vi "Remove Device.vi"(8 "error in (no error)":errorcluster, 10 "Key":T1, 11 "DeviceListPanel in":refnum<class "DeviceListPanel.lvclass">) -> (0 "error out":errorcluster, 3 "DeviceListPanel out":refnum<class "DeviceListPanel.lvclass">)   [LabVIEW 2020, in "PicoG-App.lvlib" / "DeviceListPanel.lvclass"]
uses:
  DeviceListPanel.lvclass
  DeviceListPanel.lvclass/DeviceListPanel.ctl
  Device/Device Key.ctl
  Device/Device.lvclass
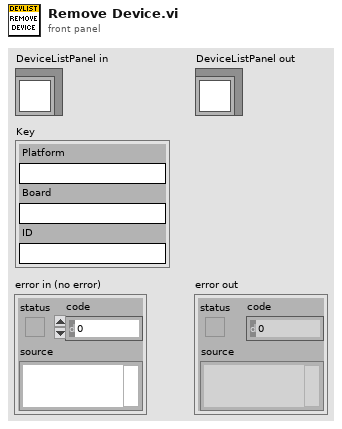
[diagram p1: front panel]
types:
  T1 = typedef "PicoG-App.lvlib/Device.lvclass/Device Key.ctl" = cluster{"Platform":string, "Board":string, "ID":string}
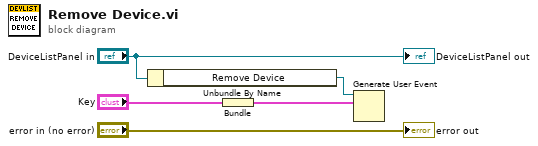
[diagram p0: block diagram]
diagram:
  n1 = Unbundle By Name("DeviceListPanel in") -> ("Remove Device"=w3:refnum<user-event>)
  n2 = Bundle("Key"="Key") -> (w1:cluster{"Key":T1})  [unwired: 1 in]
  n3 = Generate User Event(user event=w3, event data cluster=w1) -> ()  [unwired: 2 in, 2 out]
  "error out" <- "error in (no error)"
  "DeviceListPanel out" <- "DeviceListPanel in"
